vi "filter tags available for mapping to channel.vi"(10 "action channel to map to":refnum<class "TBM channel.lvclass">, 11 "engine configuration in":refnum<class "base TBM sequencer configuration.lvclass">) -> (2 "filtered seq channels":refnum<class "TBM channel.lvclass">[](array[class]), 3 "engine configuration out":refnum<class "base TBM sequencer configuration.lvclass">)   [LabVIEW 2014, in "base TBM sequencer configuration.lvclass"]
uses:
  base TBM sequencer configuration.lvclass
  <vilib>/NI/Tag Bus Module Framework/channel/TBM channel.lvclass
  <vilib>/NI/Tag Bus Module Framework/channel/TBM channel.lvclass/TBM channel.ctl
  base TBM sequencer configuration.lvclass/base TBM sequencer configuration.ctl
  <vilib>/NI/Tag Bus/tag/tag descriptor.lvclass/tag descriptor.ctl
  <vilib>/NI/Tag Bus Module Framework/channel/Read channel classification.vi
  <vilib>/NI/Tag Bus/tag/read data type.vi
  <vilib>/NI/Tag Bus/tag/tag descriptor.lvclass
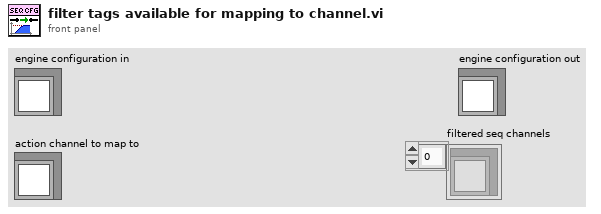
[diagram p1: front panel]
types:
  T1 = typedef "TBM channel.lvclass/channel classification.ctl" = enum16{"input data", "output data", "processing parameter", "processing result"}
  T2 = typedef "tag bus.lvlib/tag descriptor.lvclass/Data Type.ctl" = enum16{"Double", "Single", "I64", "I32", "I16", "I8", "U64", "U32", "U16", "U8", "Boolean", "String", "Array of Double", "Array of Single", "Array of I64", "Array of I32", "Array of I16", "Array of I8", "Array of U64", "Array of U32", "Array of U16", "Array of U8", "Array of Boolean", "Array of String"}
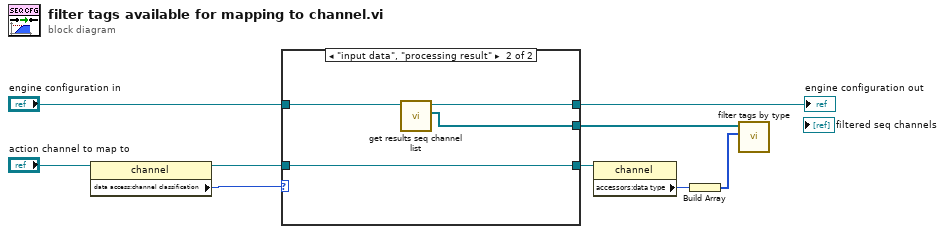
[diagram p0: block diagram]
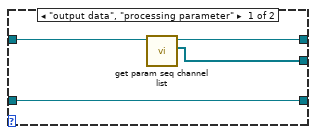
[diagram p2: hidden frame]
diagram:
  n1 = property class="channel"(reference="action channel to map to") -> (reference out=w6:refnum<class "TBM channel.lvclass">, "data access:channel classification"=w8:T1)  [unwired: 1 in, 1 out]
  n2 = case shown="\"input data\", \"processing result\"" w8 {
    tunnel: "engine configuration in" -> [w12 w16]
    tunnel: w6 -> [w13 w17]
    tunnel: [w13 w17] -> w4
    tunnel: [w11 w15] -> w5
    tunnel: [w10 w14] -> w3
    frame "output data", "processing parameter" {
      n3 = call "get param seq channel list.vi"("engine configuration in"=w12) -> ("param seq channels"=w10:refnum<class "TBM channel.lvclass">[], "engine configuration out"=w11:refnum<class "base TBM sequencer configuration.lvclass">)  [unwired: 9 in]
    }
    frame "input data", "processing result" {
      n4 = call "get results seq channel list.vi"("engine configuration in"=w16) -> ("restults seq channels"=w14:refnum<class "TBM channel.lvclass">[], "engine configuration out"=w15:refnum<class "base TBM sequencer configuration.lvclass">)  [unwired: 9 in]
    }
  }
  "engine configuration out" <- w5
  n5 = property class="channel"(reference=w4) -> ("accessors:data type"=w2:T2)  [unwired: 1 in, 2 out]
  n6 = Build Array(w2) -> (w1:T2[])
  n7 = call <vilib>:"filter tags by type.vi"("allowable types"=w1, "tags in"=w3) -> ()  [unwired: 9 in, 1 out]
